vi "Open file.vi"(9 "Nota 01":string, 10 "Sample name":string, 11 "File name":string) -> (8 "path open old":path)   [LabVIEW 2011]
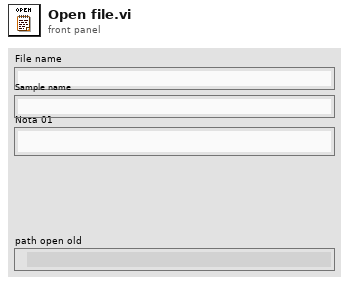
[diagram p1: front panel]
types:
  T1 = enum16{"open", "replace", "create", "open or create", "replace or create", "replace or create with confirmation"}
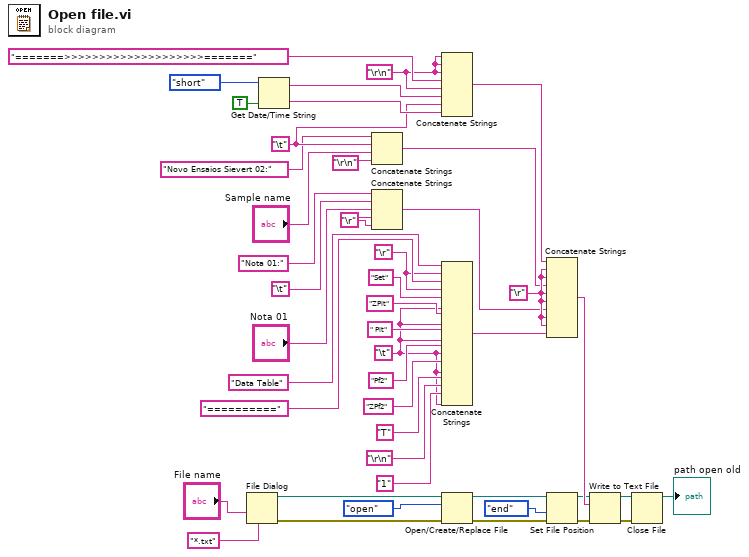
[diagram p0: block diagram]
diagram:
  w1 = "\r\n"
  w12 = "\t"
  w16 = "\r"
  w25 = "\r"
  w37 = "\r"
  w28 = "\t"
  n1 = File Dialog(6:"*.txt" ("pattern label"), 9:"File name") -> (0:w7:errorcluster, 3:w8:path)  [unwired: 2 in, 5 out]
  n2 = Get Date/Time String(date format (0)=enum16{"short", "long", "abbreviated"}."short", want seconds? (F)=TRUE) -> (date string=w41:string, time string=w40:string)  [unwired: 1 in]
  n3 = Concatenate Strings("Novo Ensaios Sievert 02:" ("string"), w28, "Sample name", "\r\n") -> (w26:string)
  n4 = Concatenate Strings("Nota 01:" ("Nota 4"), "\t", "Nota 01", w25, w25) -> (w35:string)
  n5 = Concatenate Strings(w1, w1, w1, "=======>>>>>>>>>>>>>>>>>>>>=======" ("string"), w1, w41, w28, w40) -> (w38:string)
  n6 = Concatenate Strings("Data Table" ("string"), w16, "==========" ("string"), w16, "Set" ("string"), w12, "ZPit" ("string"), w12, " Pit" ("string"), w12, "Pf2" ("string"), w12, "ZPf2" ("string"), w12, "T" ("string"), "\r\n", "1" ("string"), w12) -> (w11:string)
  n7 = Open/Create/Replace File(file path (use dialog)=w8, error in=w7, operation (0:open)=T1."open") -> (refnum out=w4:refnum<file>, error out=w9:errorcluster)  [unwired: 1 in, 3 out]
  n8 = Concatenate Strings(w38, w37, w37, w26, w37, w37, w35, w37, w37, w11) -> (w39:string)
  n9 = Set File Position(refnum=w4, from (0:start)=enum16{"start", "end", "current"}."end", error in=w9) -> (refnum out=w6:refnum<file>, error out=w5:errorcluster)  [unwired: 1 in]
  n10 = Write to Text File(file (use dialog)=w6, text=w39, error in=w5) -> (refnum out=w34:refnum<file>, error out=w31:errorcluster)  [unwired: 1 in, 1 out]
  n11 = Close File(refnum=w34, error in=w31) -> (path=→"path open old":path)  [unwired: 1 out]
